vi "Read Eulogy Bookmarks.vi"(8 "Error In":errorcluster, 11 "State In":T1) -> (0 "Error Out":errorcluster, 3 "State Out":T1)   [LabVIEW 2017, in "Bookmark Manager.lvlib"]
uses:
  Bookmark Manager.lvlib
  Controls/State.ctl
  Controls/VI Bookmark.ctl
  Controls/VI Information.ctl
  Controls/Application Information.ctl
  Controls/Bookmarks Groups.ctl
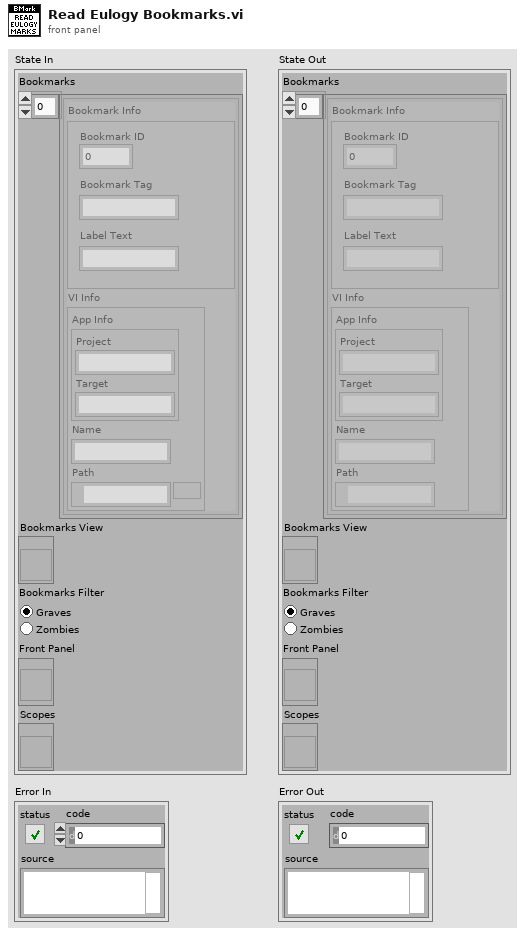
[diagram p1: front panel]
types:
  T1 = typedef "Bookmark Manager.lvlib/State.ctl" = cluster{"Bookmarks":T2[], "Bookmarks View":refnum<vi>, "Bookmarks Filter":T5, "Front Panel":refnum<vi>, "Scopes":refnum<vi>}
  T2 = typedef "Bookmark Manager.lvlib/VI Bookmark.ctl" = cluster{"Bookmark Info":cluster{"Bookmark ID":u32, "Bookmark Tag":string, "Label Text":string}, "VI Info":T3}
  T3 = typedef "Bookmark Manager.lvlib/VI Information.ctl" = cluster{"App Info":T4, "Name":string, "Path":path}
  T4 = typedef "Bookmark Manager.lvlib/Application Information.ctl" = cluster{"Project":string, "Target":string}
  T5 = typedef "Bookmark Manager.lvlib/Bookmarks Groups.ctl" = enum32{"Graves", "Zombies"}
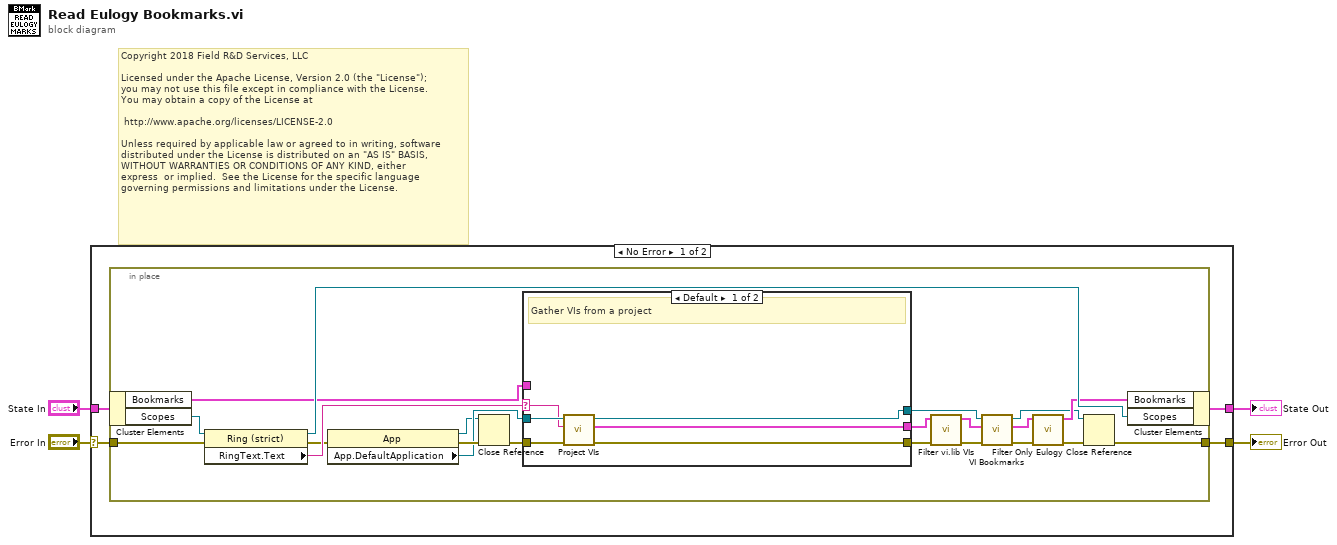
[diagram p0: block diagram]
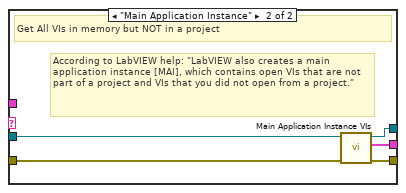
[diagram p2: hidden frame]
diagram:
  # "Copyright 2018 Field R&D Services, LLC\n\nLicensed under the Apache License, Version 2.0 (the \"License\");\nyou may not use this file except in compliance with the License.\nYou may obtain a copy of the License at\n\n\thttp://www.apache.org/licenses/LICENSE-2.0\n\nUnless required by applicable law or agreed to in writing, software\ndistributed under the License is distributed on an \"AS IS\" BASIS,\nWITHOUT WARRANTIES OR CONDITIONS OF ANY KIND, either \nexpress  or implied.  See the License for the specific language \ngoverning permissions and limitations under the License."
  n1 = case shown="No Error" "Error In" {
    selector: "Error In" -> [w5 w41]
    tunnel: [w8 w42] -> w4
    tunnel: [w7 w41] -> w3
    tunnel: "State In" -> [w6 w42]
    frame No Error {
      n2 = in-place {
        in-place-border: w5 -> [w29]
        in-place-border: [w10] -> w7
        n3 = in-place-cluster #1(w6) -> ("Bookmarks"=w25:T2[], "Scopes"=w28:refnum<vi>)
        n4 = property class="Ring (strict)"(reference=w28, error in=w29) -> (reference out=w26:refnum<vi>, error out=w15:errorcluster, "RingText.Text"=w27:string)
        n5 = property class="App"(error in=w15) -> (reference out=w11:refnum<vi>, error out=w14:errorcluster, "App.DefaultApplication"=w13:refnum<vi>)  [unwired: 1 in]
        n6 = Close Reference(reference=w11, error in (no error)=w14) -> (error out=w12:errorcluster)
        n7 = case shown="Default" w27 {
          selector: w27 -> [w30 _]
          tunnel: w25 -> [_ _]
          tunnel: w12 -> [w35 w40]
          tunnel: w13 -> [w34 w39]
          tunnel: [w31 w37] -> w20
          tunnel: [w32 w38] -> w16
          tunnel: [w33 w36] -> w17
          frame Default {
            # "Gather VIs from a project"
            n8 = call "Project VIs.vi"("Error In"=w35, "Project Name"=w30, "App In"=w34) -> ("Error Out"=w31:errorcluster, "VIs"=w33:T3[], "App Out"=w32:refnum<vi>)  [unwired: 6 in]
          }
          frame "Main Application Instance" {
            # "According to LabVIEW help: \"LabVIEW also creates a main application instance [MAI], which contains open VIs that are not part of a project and VIs that you did not open from a project.\""
            # "Get All VIs in memory but NOT in a project"
            n9 = call "Main Application Instance VIs.vi"("Error In"=w40, "App In"=w39) -> ("Error Out"=w37:errorcluster, "VIs"=w36:T3[], "App Out"=w38:refnum<vi>)  [unwired: 7 in]
          }
        }
        n10 = call "Filter vi.lib VIs.vi"("Error In"=w20, "VIs In"=w17) -> ("Error Out"=w22:errorcluster, "VIs Out"=w18:T3[])  [unwired: 8 in]
        n11 = call "VI Bookmarks.vi"("Error In"=w22, "VIs"=w18, "App In"=w16) -> ("Error Out"=w23:errorcluster, "VI Bookmarks"=w19:T2[], "App Out"=w9:refnum<vi>)  [unwired: 6 in]
        n12 = call "Filter Only Eulogy.vi"("Error In"=w23, "VI Bookmarks"=w19) -> ("Error Out"=w24:errorcluster, "Eulogy Bookmarks"=w21:T2[])  [unwired: 8 in]
        n13 = Close Reference(reference=w9, error in (no error)=w24) -> (error out=w10:errorcluster)
        n14 = in-place-cluster #1("Bookmarks"=w21, "Scopes"=w26) -> (w8:T1)
      }
    }
    frame Error {
    }
  }
  "Error Out" <- w3
  "State Out" <- w4
